vi "ma.vi"(6 "decimate":i16=1024, 9 "stages":i8=1, 11 "input":i64) -> (3 "output":i64)   [LabVIEW 2010]
uses:
  <vilib>/Platform/TimedLoop/XDataNode/XDataNode.xnode
  <vilib>/Platform/TimedLoop/XDataNode/timing_clust.ctl
  <vilib>/Platform/TimedLoop/XDataNode/nitl_modes.ctl
  <vilib>/Platform/TimedLoop/XDataNode/wakeup.ctl
  <vilib>/rvi/LocalResourceManager/LocalResourceManager.xnode
  <vilib>/rvi/DataTransferAndStorage/Container/Common/niFpgaContainerState.ctl
  <vilib>/rvi/DataTransferAndStorage/Container/Common/niFpgaDataTypeControl.ctl
  <vilib>/rvi/DataTransferAndStorage/Container/Common/niFpgaContainerImplementationControl.ctl
  <vilib>/rvi/DataTransferAndStorage/Container/Common/niFpgaContainerArbitrationOptionsControl.ctl
  <vilib>/rvi/DataTransferAndStorage/Container/Common/niFpgaTransferTypeControl.ctl
  <vilib>/rvi/DataTransferAndStorage/Container/Common/niFpgaContainerInitializationParameters.ctl
  <vilib>/rvi/Memory/Memory_Types/niFpgaMemoryInterfaceConfiguration.ctl
  <vilib>/rvi/FIFO/Fifo_Types/niFpgaFifoControlLogicControl.ctl
  <vilib>/rvi/DataTransferAndStorage/Container/Common/niFpgaContainerMetaDataKey.ctl
  <vilib>/rvi/FXPMathLib/basic elements/FxpDiscreteDelay/XNode/nifxpmath_DiscreteDelay.xnode
  <vilib>/rvi/DataTransferAndStorage/Container/XNode/niFpgaContainer.xnode
  <vilib>/rvi/DataTransferAndStorage/Container/Common/niFpgaContainerGetUniqueNameForEmu.vi
  <vilib>/rvi/DataTransferAndStorage/Container/Common/niFpgaContainerSetEmuInfo.vi
  <vilib>/rvi/eio/common/nirviEmuReportErrorAndStop.vi
  <vilib>/rvi/Memory/Memory_Emulation/nirvimemoryEmulationManagerCache_GetValue.vi
  <vilib>/rvi/Memory/Memory_Emulation/nirvimemoryEmulationManagerCache_InsertValue.vi
  <vilib>/Utility/error.llb/Clear Errors.vi
  <vilib>/rvi/Memory/Memory_Emulation/nirvimemoryEmulationManagerCache_SetValue.vi
  <vilib>/Platform/TimedLoop/XDataNode/XDNodeRunTimeDep.lvlib
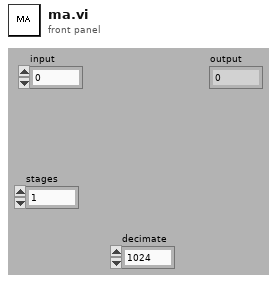
[diagram p1: front panel]
types:
  T1 = typedef "XDNodeRunTimeDep.lvlib/timing_clust.ctl" = cluster{"Expected End [f-1]":u64, "Actual End [f-1]":u64, "Finished Late? [f-1]":bool, "Expected End [i-1]":u64, "Actual End [i-1]":u64, "Finished Late? [i-1]":bool, "Expected Start [i]":u64, "Actual Start [i]":u64, "Expected Start [f]":u64, "Actual Start [f]":u64, "Source Name":string, "Structure Name":string, "Period":i64, "Deadline":i64, "Offset":i64, "Start":i64, "Priority":i32, "Timeout":i32, "Mode":T2, "Wakeup Reason":T3, "Error":errorcluster, "Source Type":string, "Secondary Source Type":string, "Global End Time":u64, "Global Start Time":u64, "Frame Duration":u64, "Iteration Duration":u64, "Assigned CPU":i32, "I/O Scan Engine Mode":u32}
  T2 = typedef "XDNodeRunTimeDep.lvlib/nitl_modes.ctl" = enum32{"No Change", "Process missed periods, maintain original phase", "Discard missed periods, maintain original phase", "Process missed periods, ignore original phase", "Discard missed periods, ignore original phase"}
  T3 = typedef "XDNodeRunTimeDep.lvlib/wakeup.ctl" = enum32{"Normal", "Aborted", "Asynchronous wakeup", "Timing source error", "Timed loop error", "Timeout"}
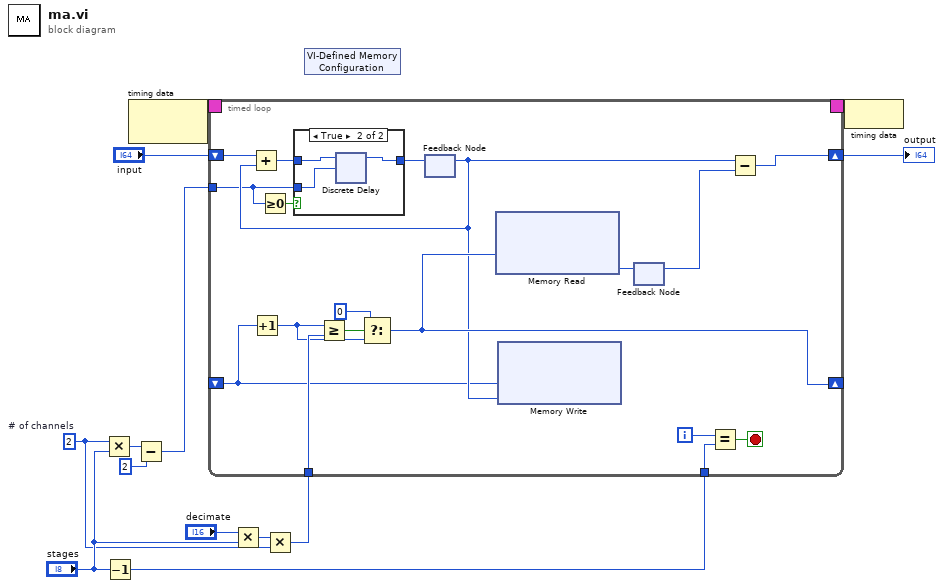
[diagram p0: block diagram]
diagram:
  w1 = i8 2  # # of channels
  n1 = Multiply(x=w1, y="stages") -> (x*y=w6:i8)
  n2 = Decrement(x="stages") -> (x-1=w8:i8)
  n3 = node-c288() -> (w13:T1)  [unwired: 1 out]
  n4 = Subtract(x=w6, y=i8 2) -> (x-y=w4:i8)
  n5 = Multiply(x="decimate", y="stages") -> (x*y=w3:i16)
  n6 = Multiply(x=w3, y=w1) -> (x*y=w2:i16)
  n7 = timed-loop {
    timing: w13 -> [_]
    timing-out: [_] -> w12
    shift-right: [w29] -> w10
    shift-left: "input" -> [w31]
    shift-right: [w21] -> _
    shift-left: _ -> [w15]
    tunnel: w8 -> [w25]
    tunnel: w2 -> [w24]
    tunnel: w4 -> [w16]
    i -> [w28]
    stop <- w27 stop-if-true
    n8 = Increment(x=w15) -> (x+1=w14:i16)
    n9 = Greater Or Equal To 0?(x=w16) -> (x >= 0?=w17:bool)
    n10 = Greater Or Equal?(x=w14, y=w24) -> (x >= y?=w23:bool)
    n11 = Select(t=i16 0, s=w23, f=w14) -> (s? t:f=w21:i16)
    n12 = feedback #1() -> (w20:i64)  [unwired: 1 out]
    n13 = Add(x=w31, y=w20) -> (x+y=w19:i64)
    n14 = case shown="True" w17 {
      tunnel: w19 -> [w283 w286]
      tunnel: [w283 w285] -> w18
      tunnel: w16 -> [_ w284]
      frame False {
      }
      frame True {
        n15 = xnode "Discrete Delay"("D"=w286, "n-1[0..15]"=w284) -> ("Q"=w285:i64)
      }
    }
    n16 = feedback-in #1(w18) -> ()
    n17 = xnode ("Memory Read")("Address"=w21) -> ("Data"=w30:i64)  [unwired: 1 in, 1 out]
    n18 = xnode ("Memory Write")("Address"=w15, "Data"=w20) -> ()  [unwired: 1 in, 1 out]
    n19 = feedback-in #2(w30) -> ()
    n20 = feedback #2() -> (w26:i64)  [unwired: 1 out]
    n21 = Equal?(x=w28, y=w25) -> (x = y?=w27:bool)
    n22 = Subtract(x=w20, y=w26) -> (x-y=w29:i64)
  }
  "output" <- w10
  n23 = xnode "VI-Defined Memory Configuration"() -> ()  [unwired: 1 out]
  n24 = node-c288(w12) -> ()
